vi "Load Recipe.vi"(8 "error in (no error)":errorcluster, 9 "Run.Start JSON":string, 10 "Recipe.lvclass":refnum<class "Recipe.lvclass">, 11 "Sequence Engine in":refnum<class "Sequence Engine.lvclass">) -> (0 "error out":errorcluster, 1 "Found?":bool, 2 "Steps Array":refnum<class "Test Step.lvclass">[](array[class]), 3 "Sequence Engine out":refnum<class "Sequence Engine.lvclass">)   [LabVIEW 2021, in "Sequence Engine.lvlib" / "Sequence Engine.lvclass"]
uses:
  Sequence Engine.lvclass
  Test Step/Test Step.lvclass
  PPLs/Recipe.lvlibp/Classes/Recipe/Recipe.lvclass
  Sequence Engine.lvclass/Sequence Engine.ctl
  Step Factory/Test Config.ctl
  Step Factory/Test Factory.lvclass
  Sequence Engine.lvlib
  MQTT Bridge/MQTT Bridge.lvlib
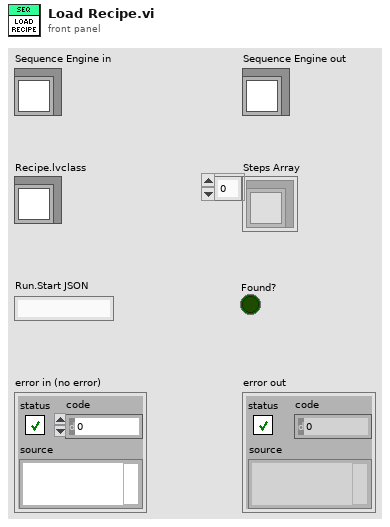
[diagram p1: front panel]
types:
  T1 = typedef "Sequence Engine.lvlib/Test Factory.lvclass/Test Config.ctl" = cluster{"Test ID":string, "Test Name":string, "Test Group":string, "Enabled?":bool, "Timeout (s)":u16, "Retry Count":u16, "Recipe Parameters":string, "Sequence Config":string}
  T2 = typedef "Recipe.lvlibp/Recipe.lvclass/Fixed Parameters.ctl" = cluster{"Test Id":string, "Test Name":string, "Test Group":string, "Timeout (s)":u16, "Retry Count":u16, "Enabled":bool}
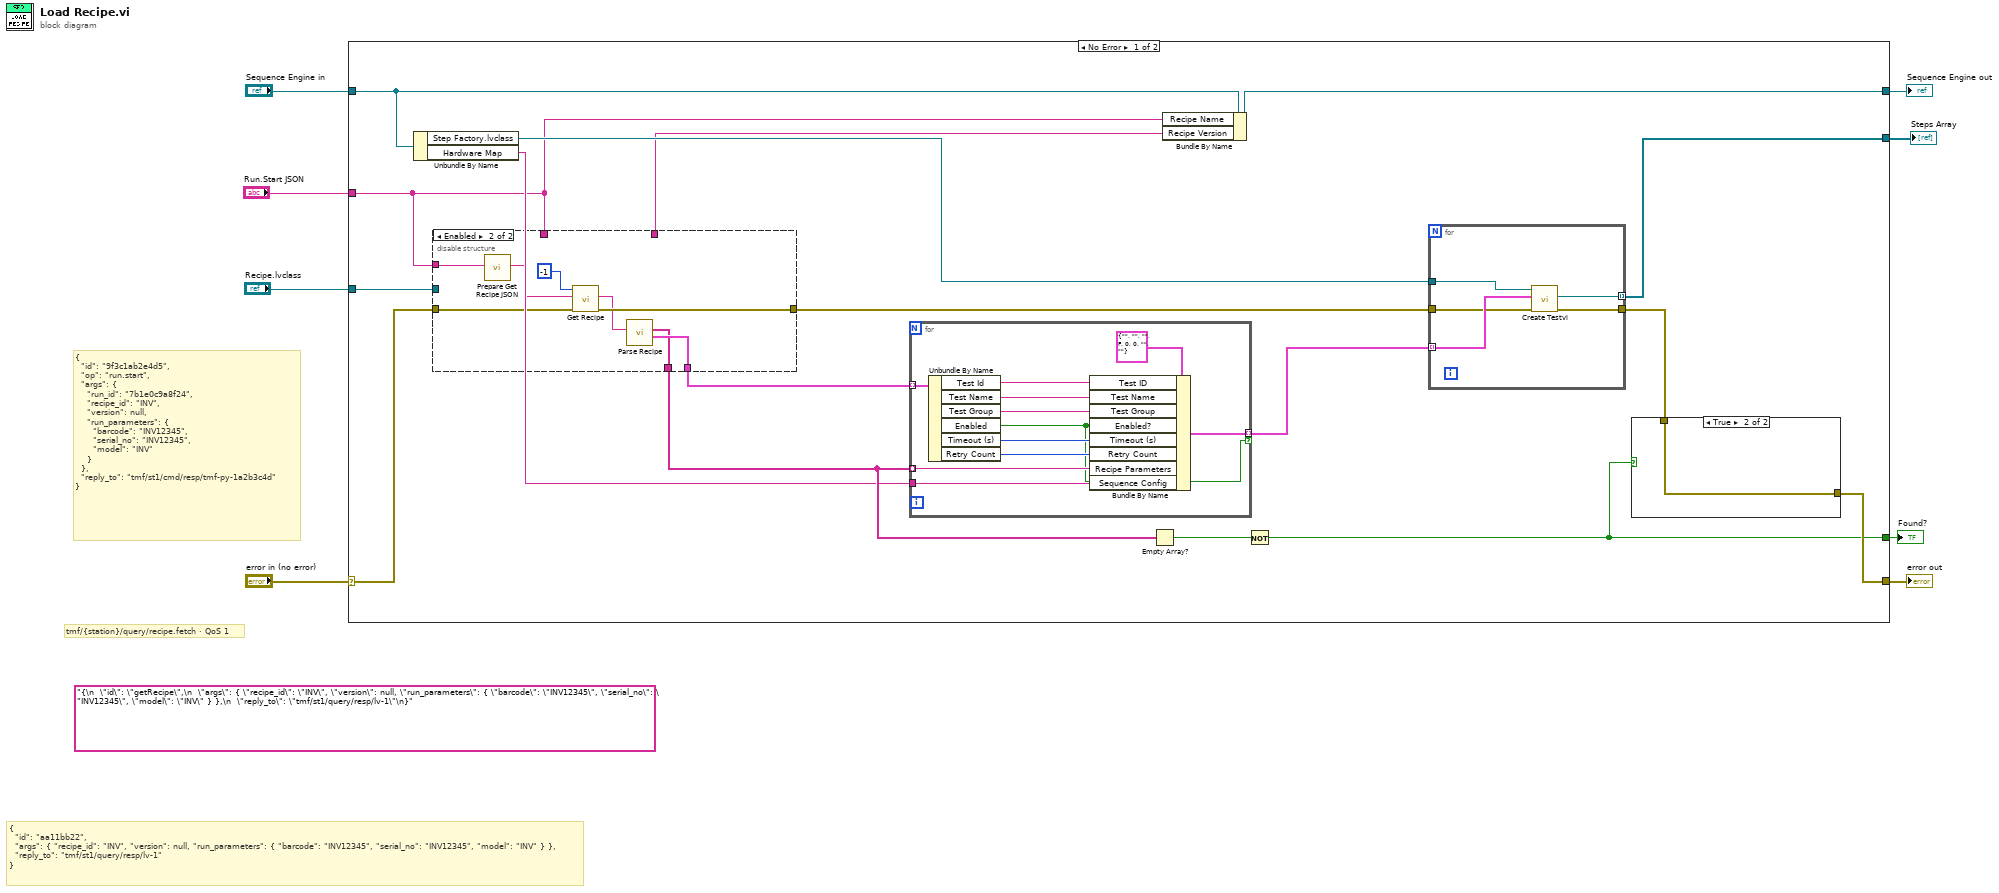
[diagram p0: block diagram]
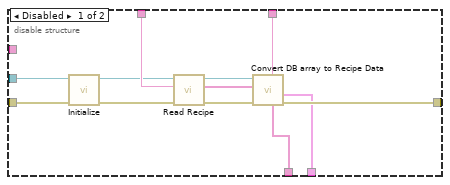
[diagram p2: hidden frame]
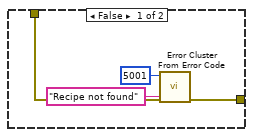
[diagram p3: hidden frame]
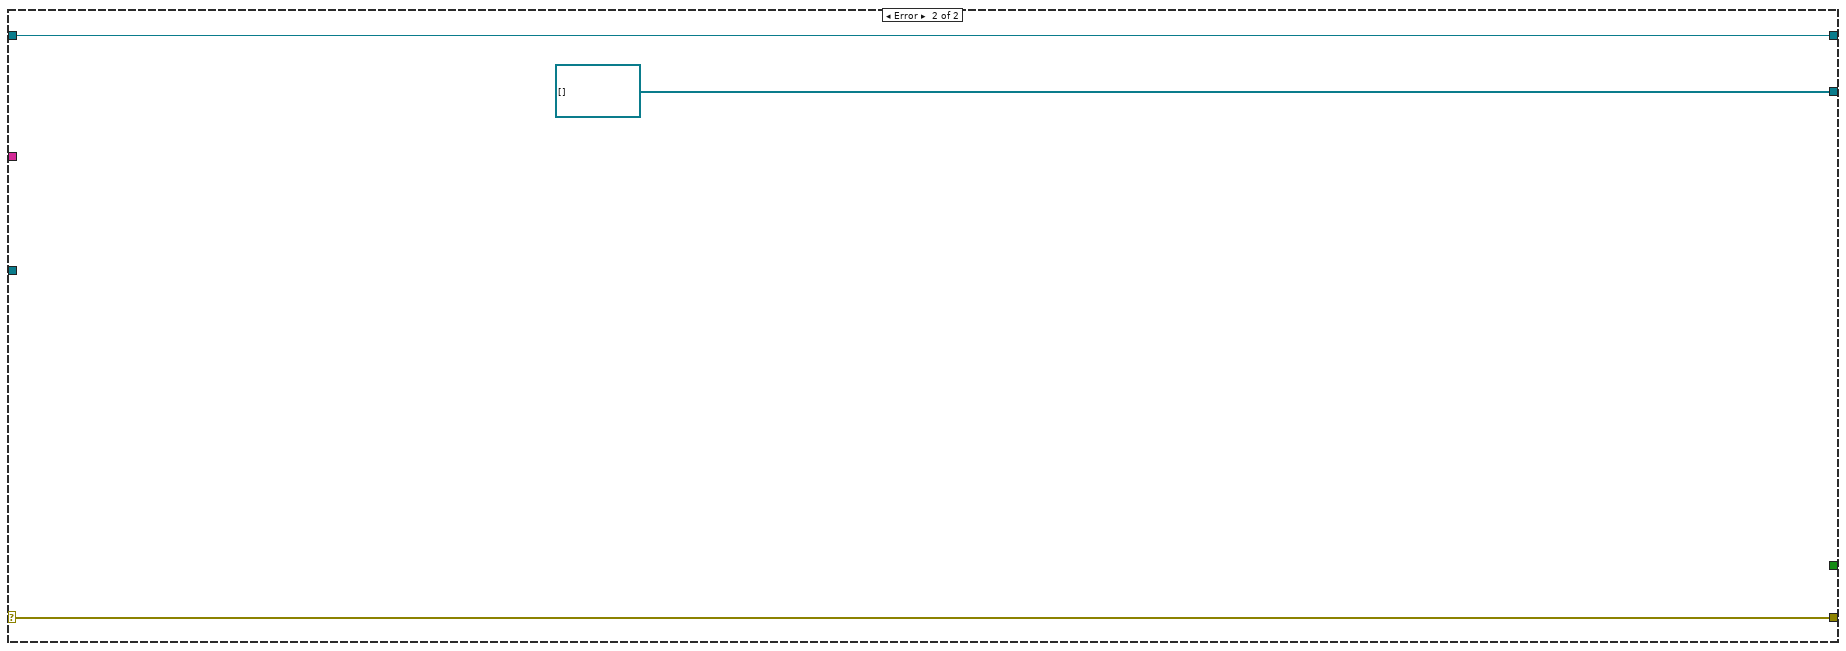
[diagram p4: hidden frame]
diagram:
  (unwired) "{\n  \"id\": \"getRecipe\",\n  \"args\": { \"recipe_id\": \"INV\", \"version\": null, \"run_parameters\": { \"barcode\": \"INV12345\", \"serial_no\": \"INV12345\", \"model\": \"INV\" } },\n  \"reply_to\": \"tmf/st1/query/resp/lv-1\"\n}"
  # "tmf/{station}/query/recipe.fetch · QoS 1"
  # "{\n  \"id\": \"aa11bb22\",\n  \"args\": { \"recipe_id\": \"INV\", \"version\": null, \"run_parameters\": { \"barcode\": \"INV12345\", \"serial_no\": \"INV12345\", \"model\": \"INV\" } },\n  \"reply_to\": \"tmf/st1/query/resp/lv-1\"\n}"
  # "{\n  \"id\": \"9f3c1ab2e4d5\",\n  \"op\": \"run.start\",\n  \"args\": {\n    \"run_id\": \"7b1e0c9a8f24\",\n    \"recipe_id\": \"INV\",\n    \"version\": null,\n    \"run_parameters\": {\n      \"barcode\": \"INV12345\",\n      \"serial_no\": \"INV12345\",\n      \"model\": \"INV\"\n    }\n  },\n  \"reply_to\": \"tmf/st1/cmd/resp/tmf-py-1a2b3c4d\"\n}"
  n1 = case shown="No Error" "error in (no error)" {
    selector: "error in (no error)" -> [w19 w69]
    tunnel: [w17 w69] -> w7
    tunnel: [w20 w68] -> w5
    tunnel: "Sequence Engine in" -> [w25 w68]
    tunnel: [w23 refnum<class "Test Step.lvclass">[] []] -> w4
    tunnel: "Recipe.lvclass" -> [w15 _]
    tunnel: "Run.Start JSON" -> [w9 _]
    tunnel: [w16 _] -> w1
    frame No Error {
      n2 = Unbundle By Name(w25) -> ("Step Factory.lvclass"=w24:refnum<class "Test Factory.lvclass">, "Hardware Map"=w10:string)
      n3 = disable-structure shown="Enabled" {
        disable-tunnel: w19 -> [w36 w41]
        disable-tunnel: w9 -> [w35 _]
        disable-tunnel: w15 -> [w32 _]
        disable-tunnel: [w31 w42] -> w14
        disable-tunnel: [w28 _] -> w13
        disable-tunnel: [w27 w39] -> w12
        disable-tunnel: [w26 w38] -> w11
        disable-tunnel: w9 -> [_ w45]
        frame Disabled {
          n4 = call "Initialize.vi"("error in (no error)"=w36, "Recipe in"=w32) -> ("error out"=w34:errorcluster, "Recipe out"=w33:refnum<class "Recipe.lvclass">)  [unwired: 8 in]
          n5 = call "Read Recipe.vi"("error in (no error)"=w34, "Recipe Name"=w35, "Recipe in"=w33) -> ("error out"=w37:errorcluster, "Recipe Data"=w29:string[], "Recipe out"=w30:refnum<class "Recipe.lvclass">)  [unwired: 6 in]
          n6 = call "Convert DB array to Recipe Data.vi"("error in (no error)"=w37, "Recipe Data"=w29, "Recipe in"=w30) -> ("error out"=w31:errorcluster, "Fixed Parameters out"=w27:T2[], "Test Parameters"=w26:string[], "Version"=w28:string)  [unwired: 3 in, 2 out]
        }
        frame Enabled {
          n7 = call "Prepare Get Recipe JSON.vi"("Run.Start JSON"=w45) -> ("resulting string"=w43:string)  [unwired: 10 in]
          n8 = call "Get Recipe.vi"("error in"=w41, "Get Recipe JSON"=w43, "Module ID"=-1) -> ("error out"=w42:errorcluster, "Get Recipe reply JSON"=w40:string)  [unwired: 6 in, 1 out]
          n9 = call "Parse Recipe.vi"("Get Recipe reply JSON"=w40) -> ("Array"=w39:T2[], "Recipe"=w38:string[])  [unwired: 9 in]
        }
      }
      n10 = for {
        tunnel: w11 -> [w59] mode=indexing
        tunnel: [w60] -> w21 mode=indexing if=w52
        tunnel: w12 -> [w58] mode=indexing
        tunnel: w10 -> [w51]
        n11 = Unbundle By Name(w58) -> ("Test Id"=w57:string, "Test Name"=w56:string, "Test Group"=w55:string, "Enabled"=w52:bool, "Timeout (s)"=w54:u16, "Retry Count"=w53:u16)
        n12 = Bundle By Name(cluster=T1 {"Test ID"="", "Test Name"="", "Test Group"="", "Enabled?"=FALSE, "Timeout (s)"=0, "Retry Count"=0, "Recipe Parameters"="", "Sequence Config"=""} ("Step Config"), "Test ID"=w57, "Test Name"=w56, "Test Group"=w55, "Enabled?"=w52, "Timeout (s)"=w54, "Retry Count"=w53, "Recipe Parameters"=w59, "Sequence Config"=w51) -> (w60:T1)
      }
      n13 = Empty Array?(array=w11) -> (empty?=w18:bool)
      n14 = Bundle By Name(cluster=w25, "Recipe Name"=w9, "Recipe Version"=w13) -> (w20:refnum<class "Sequence Engine.lvclass">)
      n15 = Not(x=w18) -> (.not. x?=w16:bool)
      n16 = for {
        tunnel: w24 -> [w66]
        tunnel: [w65] -> w23 mode=indexing
        tunnel: [w64] -> w22
        tunnel: w21 -> [w63] mode=indexing
        tunnel: w14 -> [w62]
        n17 = call "Create Testvi.vi"("error in (no error)"=w62, "Step Config"=w63, "Test Factory in"=w66) -> ("error out"=w64:errorcluster, "Test Step.lvclass"=w65:refnum<class "Test Step.lvclass">)  [unwired: 6 in, 1 out]
      }
      n18 = case shown="True" w16 {
        tunnel: w22 -> [w49 w50]
        tunnel: [w48 w50] -> w17
        frame False {
          n19 = call <vilib>:"Error Cluster From Error Code.vi"("error in (no error)"=w49, "error message (\"\")"="Recipe not found" ("error message (\"\")"), "error code (0)"=5001) -> ("error out"=w48:errorcluster)  [unwired: 6 in]
        }
        frame True {
        }
      }
    }
    frame Error {
    }
  }
  "error out" <- w7
  "Sequence Engine out" <- w5
  "Steps Array" <- w4
  "Found?" <- w1
